vi "Control Value From Registry.vi"(4 "Registry Variant Accessor (optional)":refnum<class "CConfig Variant Accessor.lvclass">, 6 "Controls":refnum<vi>[](array[refnum]), 7 "Registry Control Reference Accessor (optional)":refnum<class "Registry Ctrl Ref Accessor.lvclass">, 8 "error in (no error)":errorcluster, 9 "Use LV Default? [F]":bool, 10 "Signalling? [F]":bool, 11 "Registry Object in":refnum<class "Carya Config.lvclass">) -> (0 "error out":errorcluster, 1 "Used controls":refnum<vi>[](array[refnum]), 3 "Registry Object out":refnum<class "Carya Config.lvclass">)   [LabVIEW 2013, in "Carya Config.lvclass"]
doc: "Copyright 2018, Carya Automatisering, Wiebe Walstra."
uses:
  Carya Config.lvclass
  CConfig Ctrl Ref Accessor/Registry Ctrl Ref Accessor.lvclass
  CConfig Variant Accessor/CConfig Variant Accessor.lvclass
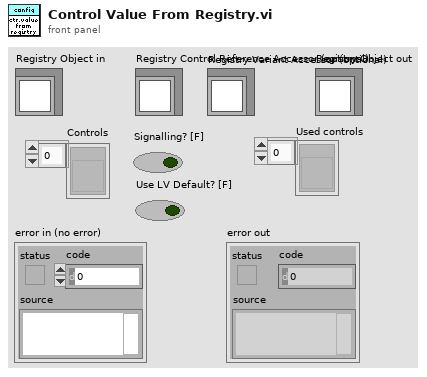
[diagram p1: front panel]
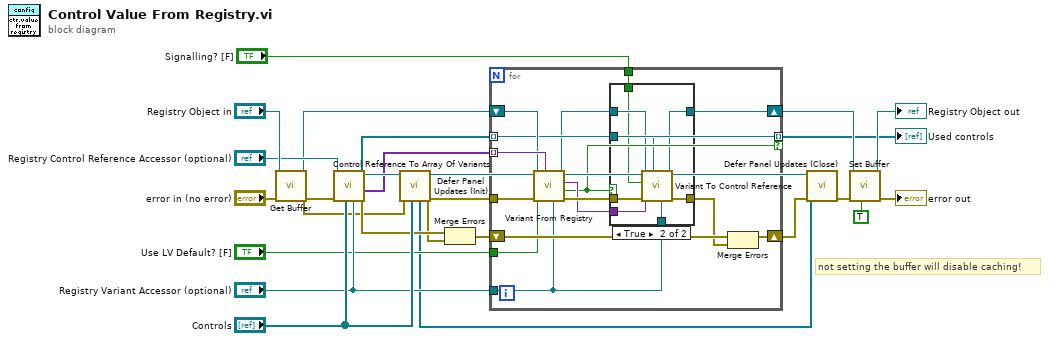
[diagram p0: block diagram]
diagram:
  # "not setting the buffer will disable caching!"
  n1 = call-dynamic "Get Buffer.vi"("error in (no error)"="error in (no error)", "Carya Config in"="Registry Object in") -> ("error out"=w3:errorcluster, "Config"=w9:refnum<class "Carya Config.lvclass">)  [unwired: 8 in]
  n2 = call-dynamic "Control Reference To Array Of Variants.vi"("Registry Variant Accessor"="Registry Variant Accessor (optional)", "Controls"="Controls", "error in (no error)"=w3, "Registry Control Reference Accessor in"="Registry Control Reference Accessor (optional)") -> ("error out"=w7:errorcluster, "Variants"=w17:variant[], "Controls"=w12:refnum<vi>[], "Registry Control Reference Accessor out"=w18:refnum<class "Registry Ctrl Ref Accessor.lvclass">)  [unwired: 4 in]
  n3 = call-dynamic "Defer Panel Updates (Init).vi"("Controls"="Controls", "error in (no error)"=w3, "Registry Control Reference Accessor in"=w18) -> ("error out"=w6:errorcluster, "Registry Control Reference Accessor out"=w13:refnum<class "Registry Ctrl Ref Accessor.lvclass">, "Panel refs"=w5:refnum<vi>[])  [unwired: 6 in]
  n4 = Merge Errors(w7, w6) -> (w8:errorcluster)
  n5 = for {
    tunnel: w6 -> [w39]
    tunnel: w17 -> [w38] mode=indexing
    tunnel: "Registry Variant Accessor (optional)" -> [w26]
    shift-right: [w36] -> w14
    shift-left: w8 -> [w37]
    shift-right: [w27] -> w10
    shift-left: w9 -> [w31]
    tunnel: w12 -> [w30] mode=indexing
    tunnel: "Use LV Default? [F]" -> [w32]
    tunnel: [w30] -> w4 mode=indexing if=w29
    tunnel: "Signalling? [F]" -> [w25]
    n6 = call "Variant From Registry.vi"("Registry Variant Accessor in"=w26, "Variant"=w38, "error in (no error)"=w39, "Use LV Default? [F]"=w32, "Carya Config in"=w31) -> ("error out"=w35:errorcluster, "Set?"=w29:bool, "Variant"=w33:variant, "Carya Config out"=w28:refnum<class "Carya Config.lvclass">)  [unwired: 3 in]
    n7 = case shown="True" w29 {
      tunnel: w35 -> [w41 w49]
      tunnel: [w41 w48] -> w34
      tunnel: w30 -> [_ w47]
      tunnel: w33 -> [_ w46]
      tunnel: w28 -> [w40 w45]
      tunnel: [w40 w44] -> w27
      tunnel: w26 -> [_ w43]
      tunnel: w25 -> [_ w42]
      frame False {
      }
      frame True {
        n8 = call-dynamic "Variant To Control Reference.vi"("Registry Variant Accessor in"=w43, "Ctl Refnum"=w47, "error in (no error)"=w49, "Value"=w46, "Signalling? [F]"=w42, "Carya Config in"=w45) -> ("error out"=w48:errorcluster, "Carya Config out"=w44:refnum<class "Carya Config.lvclass">)  [unwired: 4 in]
      }
    }
    n9 = Merge Errors(w37, w34) -> (w36:errorcluster)
  }
  "Used controls" <- w4
  n10 = call-dynamic "Defer Panel Updates (Close).vi"("error in (no error)"=w14, "Panel refs"=w5, "Registry Control Reference Accessor in"=w13) -> ("error out"=w24:errorcluster)  [unwired: 7 in, 1 out]
  n11 = call-dynamic "Set Buffer.vi"("Set? [T]"=TRUE, "error in (no error)"=w24, "Carya Config"=w10) -> ("error out"=→"error out":errorcluster, "Carya Config out"=→"Registry Object out":refnum<class "Carya Config.lvclass">)  [unwired: 7 in]
